vi "SaveControlValues.vi"(5 "Axis":T1=1 items=["Axis Control"=0, "Axis 1"=1, "Axis 2"=2, "Axis 3"=3, "Axis 4"=4, "Axis 5"=5, "Axis 6"=6, "Axis 7"=7, "Axis 8"=8, "Vector Space Control"=16, "Vector Space 1"=17, "Vector Space 2"=18, "Vector Space 3"=19, "Vector Space 4"=20, "Encoder Control"=32, "Encoder 1"=33, "Encoder 2"=34, "Encoder 3"=35, "Encoder 4"=36, "Encoder 5"=37, "Encoder 6"=38, "Encoder 7"=39, "Encoder 8"=40, "DAC Channel 1"=49, "DAC Channel 2"=50, "DAC Channel 3"=51, "DAC Channel 4"=52, "DAC Channel 5"=53, "DAC Channel 6"=54, "DAC Channel 7"=55, "DAC Channel 8"=56, "Stepper Output 1"=65, "Stepper Output 2"=66, "Stepper Output 3"=67, "Stepper Output 4"=68, "Stepper Output 5"=69, "Stepper Output 6"=70, "Stepper Output 7"=71, "Stepper Output 8"=72, "ADC Channel 1"=81, "ADC Channel 2"=82, "ADC Channel 3"=83, "ADC Channel 4"=84, "ADC Channel 5"=85, "ADC Channel 6"=86, "ADC Channel 7"=87, "ADC Channel 8"=88], 6 "error in":errorcluster, 9 "path":path) -> (0 "error out":errorcluster)   [LabVIEW 2010]
uses:
  <vilib>/Motion/FlexMotion/CustomControls/CustomControls.llb/Resource Out (Enum).flx
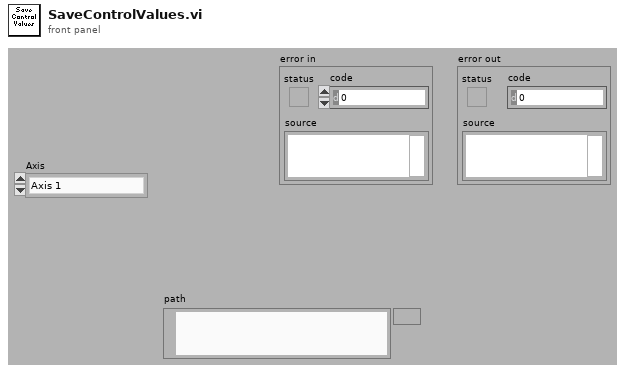
[diagram p1: front panel]
types:
  T1 = typedef "Resource Out (Enum).flx" = u16
  T2 = cluster{"Name":string, "type string":i16[], "data string":string}
  T3 = cluster{"Name":string, "type string":i16[], "data string":string}[]
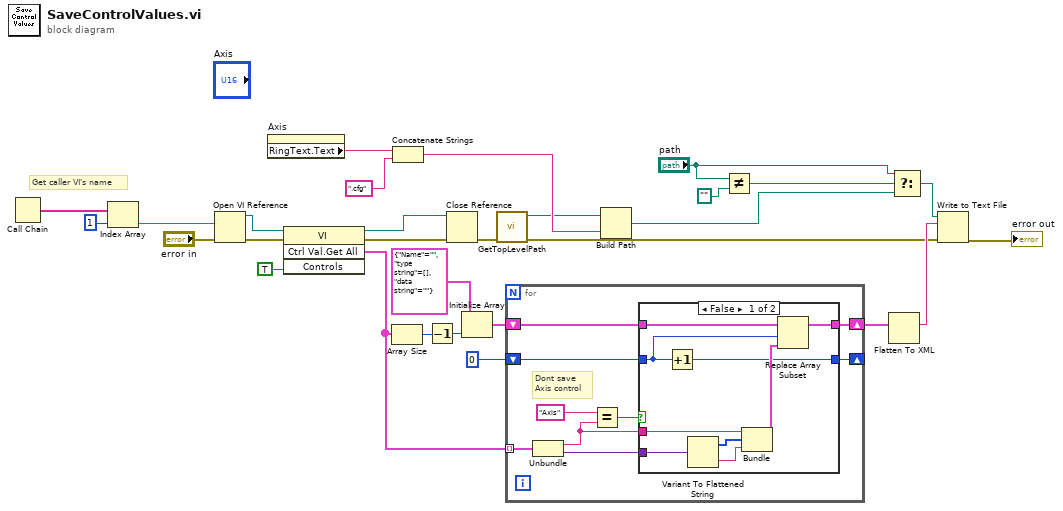
[diagram p0: block diagram]
diagram:
  # "Get caller VI's name"
  n1 = Call Chain() -> (call chain=w18:string[])
  n2 = Index Array(array=w18, index=1) -> (element=w16:string)
  n3 = Open VI Reference(vi path=w16, error in (no error)="error in") -> (vi reference=w15:refnum<vi>, error out=w11:errorcluster)  [unwired: 4 in]
  n4 = property on="Axis" class="Ring (strict)"() -> ("RingText.Text"=w8:string)  [unwired: 2 in, 2 out]
  n5 = invoke class="VI" method="Ctrl Val.Get All"(reference=w15, error in=w11, "Controls"=TRUE ("Save control values")) -> (reference out=w14:refnum<vi>, error out=w13:errorcluster, "Get All Control Values Variant"=w6:cluster{"Name":string, "Variant Data":variant}[])  [unwired: 1 in, 1 out]
  n6 = Array Size(array=w6) -> (size(s)=w2:i32)
  n7 = Concatenate Strings(w8, ".cfg" ("string")) -> (w25:string)
  n8 = Decrement(x=w2) -> (x-1=w3:i32)
  n9 = Close Reference(reference=w14, error in (no error)=w13) -> (error out=w10:errorcluster)
  n10 = Initialize Array(T2 {"Name"="", "type string"=[], "data string"=""} ("output cluster"), w3) -> (w4:T3)
  n11 = call "GetTopLevelPath.vi"("error in"=w10) -> ("error out"=w9:errorcluster, "path"=w12:path)  [unwired: 9 in]
  n12 = for {
    tunnel: w6 -> [w38] mode=indexing
    shift-right: [w34] -> w7
    shift-left: w4 -> [w33]
    shift-right: [w30] -> _
    shift-left: 0 -> [w31]
    # "Dont save\nAxis control"
    n13 = Unbundle(w38) -> ("Name"=w35:string, "Variant Data"=w37:variant)
    n14 = Equal?(x="Axis", y=w35) -> (x = y?=w36:bool)
    n15 = case shown="False" w36 {
      tunnel: w37 -> [w47 _]
      tunnel: w35 -> [w44 _]
      tunnel: [w43 w49] -> w34
      tunnel: w33 -> [w41 w49]
      tunnel: w31 -> [w40 w48]
      tunnel: [w39 w48] -> w30
      frame False {
        n16 = Increment(x=w40) -> (x+1=w39:i32)
        n17 = Variant To Flattened String(Variant=w47) -> (data string=w45:string, 1:w46:i16[])
        n18 = Bundle("Name"=w44, "type string"=w46, "data string"=w45) -> (w42:T2)  [unwired: 1 out]
        n19 = Replace Array Subset(array=w41, new element=w42, index=w40) -> (w43:T3)
      }
      frame True {
      }
    }
  }
  n20 = Build Path(base path=w12, name or relative path=w25) -> (appended path=w21:path)
  n21 = Not Equal?(x="path", y=path "") -> (x != y?=w24:bool)
  n22 = Flatten To XML(anything=w7) -> (xml string=w28:string)
  n23 = Select(t="path", s=w24, f=w21) -> (s? t:f=w20:path)
  n24 = Write to Text File(file (use dialog)=w20, text=w28, error in=w9) -> (error out=→"error out":errorcluster)  [unwired: 3 out]
